vi "Supported Smart Syntax Representation.vi"(0 "Message Popup in":refnum<class "print screen.lvclass">, 11 "error in (no error)":errorcluster) -> (4 "Message Popup out":refnum<class "print screen.lvclass">, 6 "Smart Syntax Representation List":string[](array[string]), 15 "error out":errorcluster)   [LabVIEW 2016, in "print screen.lvclass"]
uses:
  print screen.lvclass
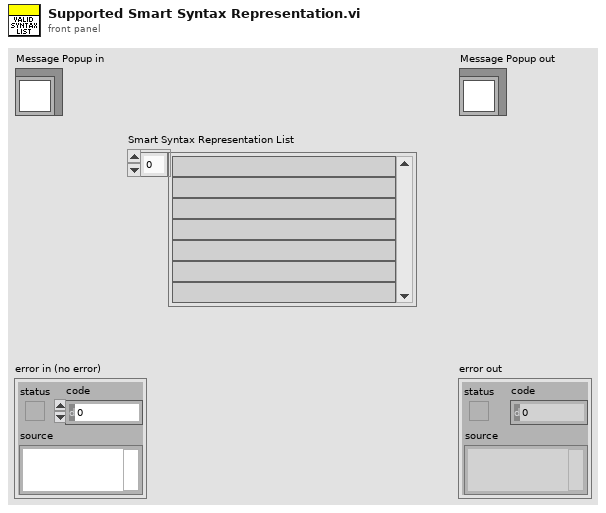
[diagram p1: front panel]
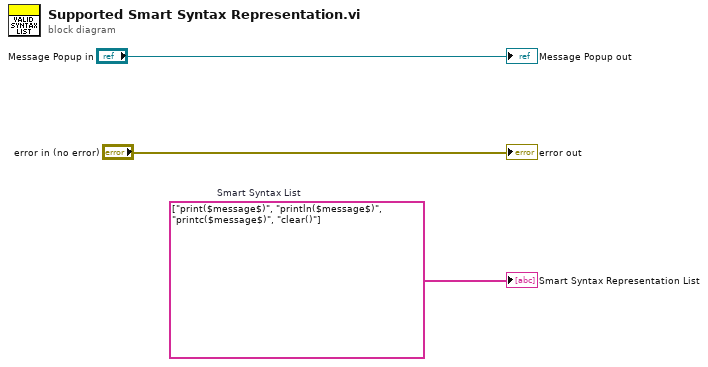
[diagram p0: block diagram]
diagram:
  w1 = string[] ["print($message$)", "println($message$)", "printc($message$)", "clear()"]  # Smart Syntax List
  "error out" <- "error in (no error)"
  "Message Popup out" <- "Message Popup in"
  "Smart Syntax Representation List" <- w1
